vi "head.vi"(7 "transmit queue":refnum<queue>, 9 "server information":T1, 10 "application request in":T2, 11 "test responder in":refnum<class "test responder.lvclass">) -> (0 "error out":errorcluster, 3 "test responder out":refnum<class "test responder.lvclass">)   [LabVIEW 2016, in "test responder.lvclass"]
uses:
  test responder.lvclass
  HTTP server/http response.ctl
  HTTP server/http response packet type.ctl
  HTTP headers/http header data.ctl
  HTTP server/http request.ctl
  HTTP server/http method.ctl
  HTTP server/http server info.ctl
  HTTP responder/http responder.lvclass
  HTTP server/Basic HTTP server.lvclass
  HTTP headers/http headers.lvlib
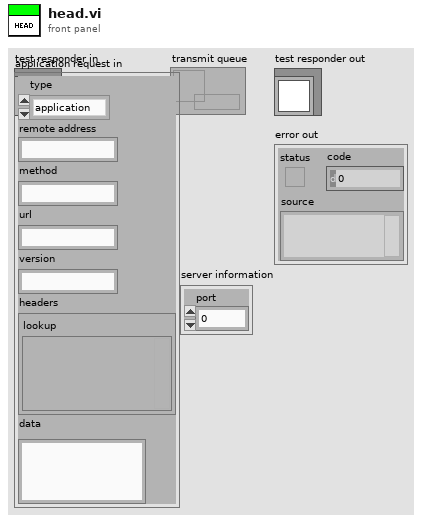
[diagram p1: front panel]
types:
  T1 = typedef "Basic HTTP server.lvclass/http server info.ctl" = cluster{"port":u16}
  T2 = typedef "Basic HTTP server.lvclass/http request.ctl" = cluster{"type":T3, "remote address":string, "method":string, "url":string, "version":string, "headers":T4, "data":string}
  T3 = typedef "Basic HTTP server.lvclass/http method.ctl" = enum16{"application", "error", "upgrade", "expect"}
  T4 = typedef "http headers.lvlib/http header data.ctl" = cluster{"lookup":variant}
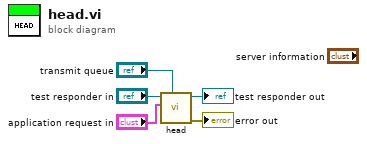
[diagram p0: block diagram]
diagram:
  n1 = call-parent "head.vi"("transmit queue"="transmit queue", "application request in"="application request in", "http responder in"="test responder in") -> ("error out"=→"error out":errorcluster, "http responder out"=→"test responder out":refnum<class "test responder.lvclass">)  [unwired: 7 in]
